vi "Waveform Generator.vi"(8 "Error In":errorcluster, 10 "amplitude":dbl, 11 "frequency":dbl) -> (0 "Error Out":errorcluster, 3 "signal out":waveform(dbl)(graph))   [LabVIEW 2023]
doc: "Use this VI as the VI under test for Waveform Generator.lvtest."
uses:
  <vilib>/measure/NI_MABase.lvlib
panel:
  # "Overview: Use this VI as the VI under test for Waveform Generator.lvtest.\nRequirements: LabVIEW Full Development System, Unit Test Framework Toolkit\nInstructions:\n1.  Execute the Waveform Generator.lvtest test file for this VI. In the Project Explorer window, expand the Unit Test Files folder, right-click Waveform Generator.lvtest, and select Run from the shortcut menu.\n2.  View the test results in the Unit Test Framework Results window, which shows that this test passes.\n3.  In the Project Explorer window, double-click Waveform Generator.lvtest to display the Test Properties dialog box.\n4.  Select Test Vectors from the Category list to display the Test Vectors page. Understand how to add a test vector file for a test.\n5.  Select Test Cases from the Category list to display the Test Cases page. Understand how to assign test vectors to input and output terminals in the VI under test.\n6.  Click OK to close the dialog box.\n7.  In the Project Explorer window, double-click waveform parameters.lvvect to display the Test Vector File Properties dialog box. Understand how to use a test vector file that includes test vector files.\n8.  Click Cancel to close the dialog box."
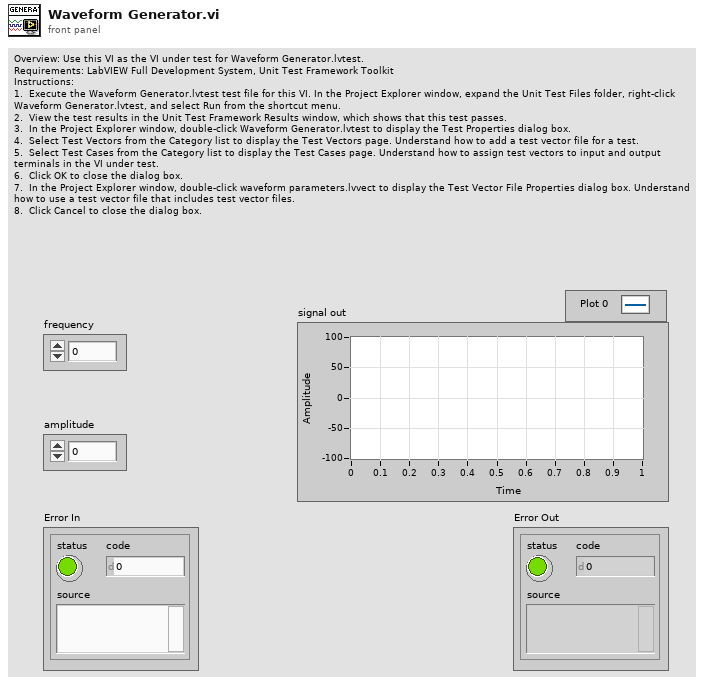
[diagram p1: front panel]
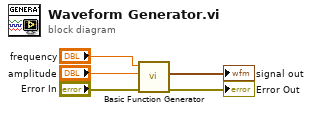
[diagram p0: block diagram]
diagram:
  n1 = call <vilib>:"Basic Function Generator.vi"("error in (no error)"="Error In", "amplitude"="amplitude", "frequency"="frequency") -> ("error out"=→"Error Out":errorcluster, "signal out"=→"signal out":waveform(dbl))  [unwired: 6 in, 1 out]
